vi "DELETE_VENDING MACHINE.vi"(8 "error in (no error)":errorcluster, 11 "USR":T1) -> (0 "error out":errorcluster)   [LabVIEW 2019, in "DB_VENDING MACHINE.lvlib"]
uses:
  DB_VENDING MACHINE.lvlib
  6 SEMESTRE/ADQUISICION_DATOS/BASE DE DATOS WEB/DB_LIBRARY/USR.ctl
  <vilib>/addons/database/NI_Database_API.lvlib
  6 SEMESTRE/ADQUISICION_DATOS/BASE DE DATOS WEB/DB_LIBRARY/DB_LIBARY.lvlib
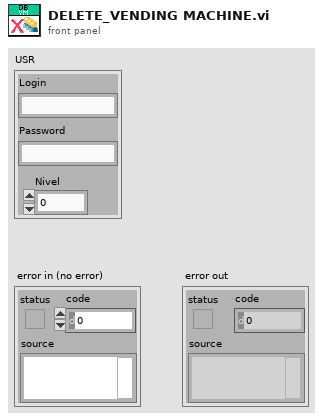
[diagram p1: front panel]
types:
  T1 = typedef "DB_LIBARY.lvlib/USR.ctl" = cluster{"Login":string, "Password":string, "Nivel":u8}
  T2 = typedef "NI_Database_API.lvlib/Conn ObjectReference.ctl" = refnum<k1>
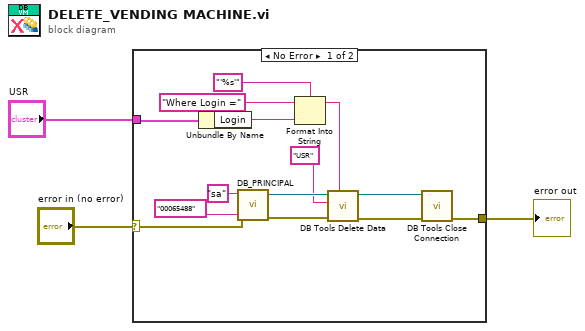
[diagram p0: block diagram]
diagram:
  n1 = case shown="No Error" "error in (no error)" {
    selector: "error in (no error)" -> [w9 w18]
    tunnel: "USR" -> [w5 _]
    tunnel: [w10 w18] -> w2
    frame No Error {
      n2 = Unbundle By Name(w5) -> ("Login"=w6:string)
      n3 = call "DB_PRINCIPAL.vi"("error in (no error)"=w9, "password"="00065488", "userID"="sa") -> ("error out"=w16:errorcluster, "connection reference"=w17:T2)  [unwired: 7 in]
      n4 = Format Into String(format string="'%s'", initial string="Where Login =" ("condition"), w6) -> (resulting string=w7:string)  [unwired: 1 in, 1 out]
      n5 = call <vilib>:"DB Tools Delete Data.vi"("condition"=w7, "error in (no error)"=w16, "table"="USR", "connection reference"=w17) -> ("error out"=w15:errorcluster, "connection reference out"=w14:T2)  [unwired: 6 in]
      n6 = call <vilib>:"DB Tools Close Connection.vi"("error in (no error)"=w15, "connection reference"=w14) -> ("error out"=w10:errorcluster)  [unwired: 5 in]
    }
    frame Error {
    }
  }
  "error out" <- w2
